vi "TDMS Write.vi"(7 "Channel Name":string, 8 "error in (no error)":errorcluster, 9 "Group Name":string, 10 "TDMS in":refnum<k34>, 11 "Path in":refnum<class "Path.lvclass">) -> (0 "error out":errorcluster, 2 "TDMS Out":refnum<k34>)   [LabVIEW 2020, in "Data.lvlib" / "Path.lvclass"]
doc: "Write Generic Data to a TDMS file."
uses:
  Path.lvclass
  Path.lvclass/Path.ctl
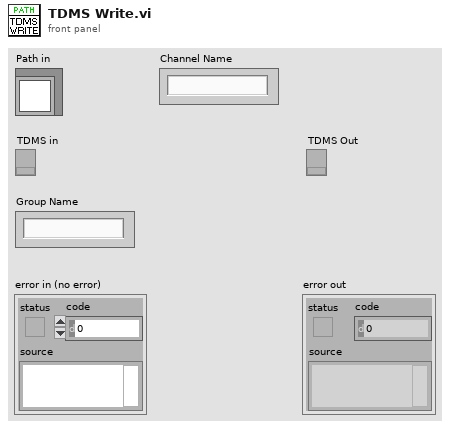
[diagram p1: front panel]
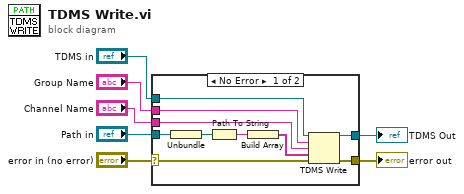
[diagram p0: block diagram]
diagram:
  n1 = case shown="No Error" "error in (no error)" {
    selector: "error in (no error)" -> [w17 w18]
    tunnel: [w16 w18] -> w1
    tunnel: "TDMS in" -> [w15 w19]
    tunnel: [w14 w19] -> w2
    tunnel: "Channel Name" -> [w13 _]
    tunnel: "Group Name" -> [w12 _]
    tunnel: "Path in" -> [w11 _]
    frame No Error {
      n2 = Unbundle(w11) -> (w9:path)
      n3 = Path To String(path=w9) -> (string=w8:string)
      n4 = Build Array(w8) -> (w10:string[])
      n5 = TDMS Write(0:w15, 5:w12, 7:w13, 9:w10, 11:w17) -> (4:w14:refnum<k34>, 15:w16:errorcluster)  [unwired: 1 in, 2 out]
    }
    frame Error {
    }
  }
  "error out" <- w1
  "TDMS Out" <- w2
